vi "Get 2614B value.vi"(11 "输出簇输入":T1 {"Instrument"."Input (0:A)" items=["A", "B"]; "Instrument"."Heater Output (1:1)" items=["1"=1, "2"=2]; "SR830+6221"."Reserve 4" items=["Auto Reserve"=-1, "High Reserve"=0, "Normal"=1, "Low Noise"=2]; "SR830+6221"."Reserve 3" items=["Auto Reserve"=-1, "High Reserve"=0, "Normal"=1, "Low Noise"=2]; "SR830+6221"."Reserve 2" items=["Auto Reserve"=-1, "High Reserve"=0, "Normal"=1, "Low Noise"=2]; "SR830+6221"."Reserve 1" items=["Auto Reserve"=-1, "High Reserve"=0, "Normal"=1, "Low Noise"=2]; "SR830+6221"."source" items=["SR830 1", "SR830 2", "SR830 3", "SR830 4"]}) -> (3 "数组":string[](array[string]))   [LabVIEW 2019, in "Get value.lvlib"]
uses:
  config.ctl
  <vilib>/NI/Modbus Library/API/Master/Modbus Master.lvclass
  initialize.ctl
  Instrument.ctl
  Instrument Type.ctl
  lib/QDInstrument.dll
  335 state.ctl
  SubVI/limit.ctl
  9T mag field stauts.ctl
  warning.ctl
  lib/Keithley 2600 Series/Public/Data/Read Measurement (Current and Voltage).vi
  SubVI/Get value.lvlib
  lib/Keithley 2600 Series/Keithley 2600 Series.lvlib
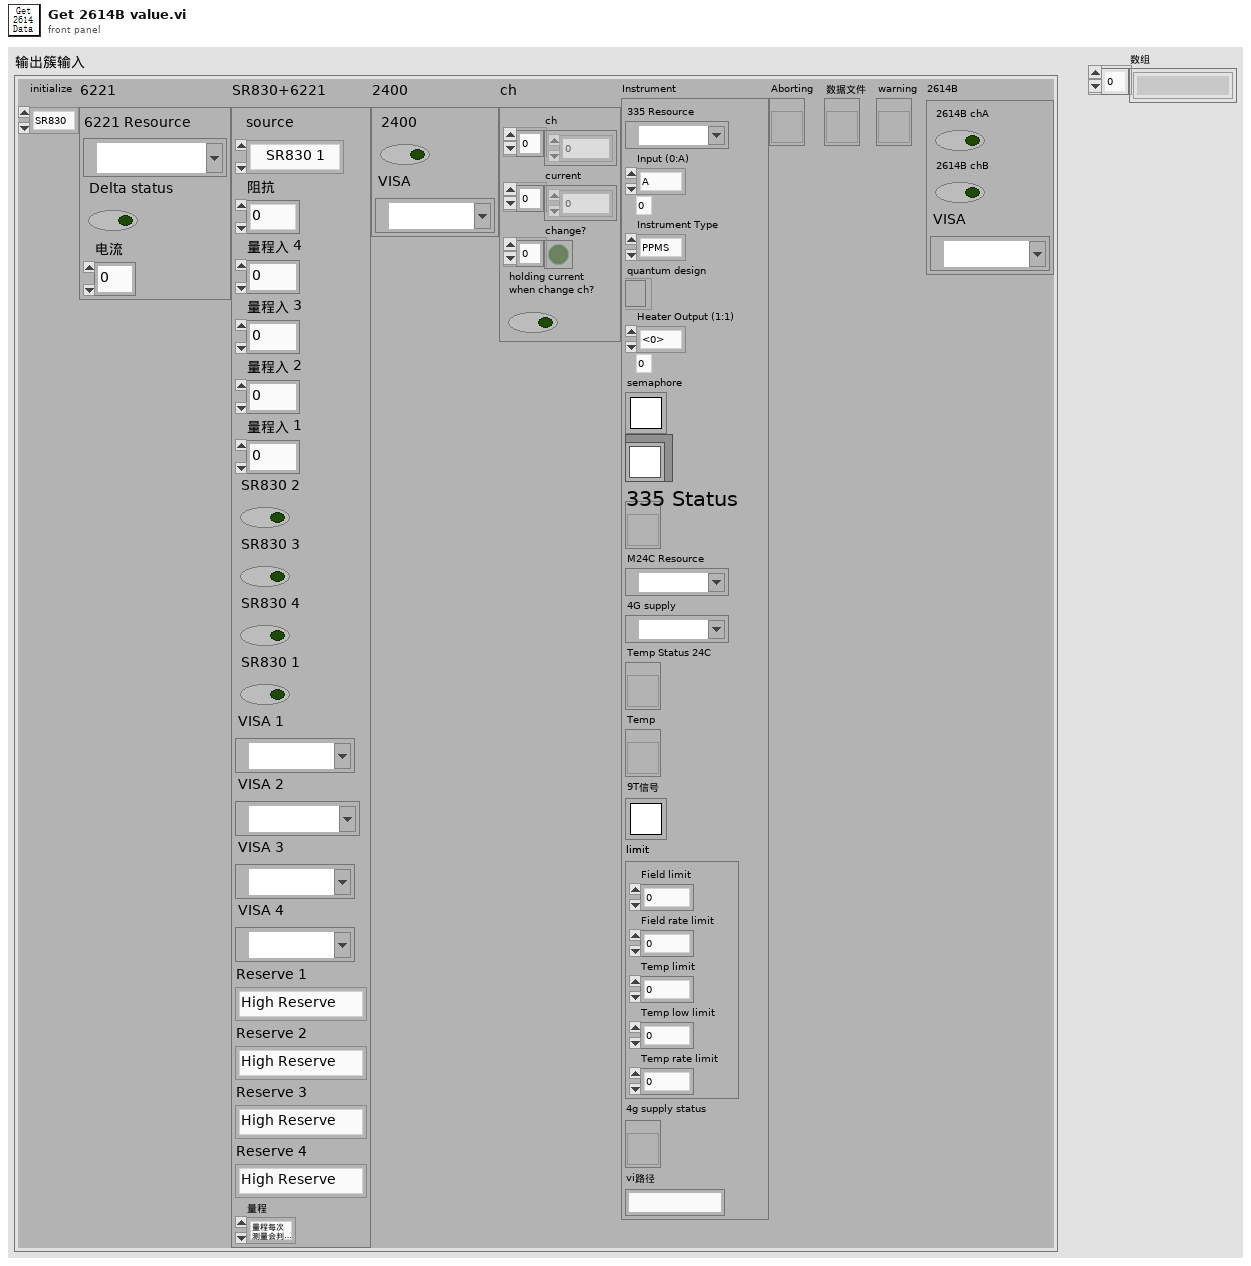
[diagram p1: front panel]
types:
  T1 = typedef "config.ctl" = cluster{"initialize":T2, "6221":cluster{"6221 Resource":refnum<visa-resource-name>, "Delta status":bool, "电流":dbl}, "SR830+6221":cluster{"source":u16, "阻抗":dbl, "量程入 4":i32, "量程入 3":i32, "量程入 2":i32, "量程入 1":i32, "SR830 2":bool, "SR830 3":bool, "SR830 4":bool, "SR830 1":bool, "VISA 1":refnum<visa-resource-name>, "VISA 2":refnum<visa-resource-name>, "VISA 3":refnum<visa-resource-name>, "VISA 4":refnum<visa-resource-name>, "Reserve 1":i16, "Reserve 2":i16, "Reserve 3":i16, "Reserve 4":i16, "量程":enum16{"量程每次测量会判定", "量程不变为设定值"}}, "2400":cluster{"2400":bool, "VISA":refnum<visa-resource-name>}, "ch":cluster{"ch":i32[], "current":dbl[], "change?":bool[], "holding current\nwhen change ch?":bool}, "Instrument":T3, "Aborting":refnum<vi>, "数据文件":refnum<vi>, "warning":refnum<vi>, "2614B":cluster{"2614B chA":bool, "2614B chB":bool, "VISA":refnum<visa-resource-name>}}
  T2 = typedef "initialize.ctl" = enum16{"SR830", "keithley6221-SR830", "Delta", "Delta-tunnelling", "keithley6221-2182-DC"}
  T3 = typedef "Instrument.ctl" = cluster{"335 Resource":refnum<visa-resource-name>, "Input (0:A)":u16, "Instrument Type":T4, "quantum design":refnum<k24>, "Heater Output (1:1)":u16, "semaphore":T5, "TCP master instance":refnum<class "Modbus Master.lvclass">, "335 Status":refnum<vi>, "M24C Resource":refnum<visa-resource-name>, "4G supply":refnum<visa-resource-name>, "Temp Status 24C":refnum<vi>, "Temp":refnum<vi>, "9T信号":T5, "limit":T6, "4g supply status":refnum<vi>, "vi路径":string}
  T4 = typedef "Instrument Type.ctl" = enum16{"PPMS", "VersaLab", "DynaCool", "SVSM", "PPMS-Rotate", "Lakeshore335", "9T mag"}
  T5 = typedef "Semaphore RefNum" = refnum<k1>
  T6 = typedef "limit.ctl" = cluster{"Field limit":dbl, "Field rate limit":dbl, "Temp limit":dbl, "Temp low limit":dbl, "Temp rate limit ":dbl}
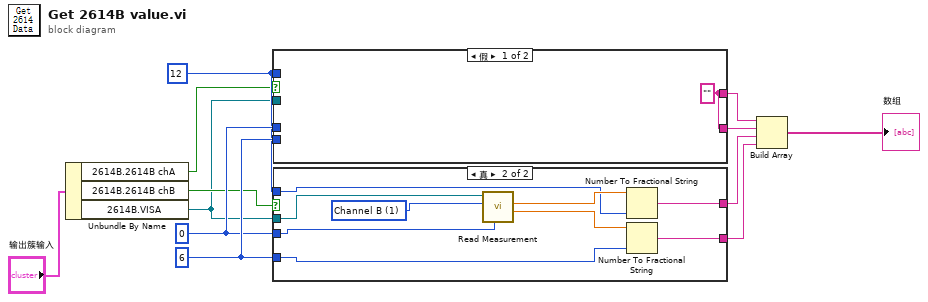
[diagram p0: block diagram]
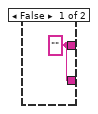
[diagram p2: hidden frame]
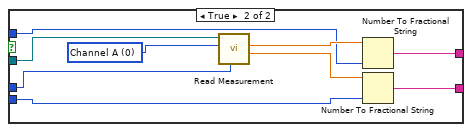
[diagram p3: hidden frame]
diagram:
  w6 = 0 ("Wait Time (10 S)")
  w5 = i16 12 ("精度(6)")
  w7 = i16 6 ("精度(6)")
  n1 = Unbundle By Name("输出簇输入") -> ("2614B.2614B chA"=w2:bool, "2614B.2614B chB"=w4:bool, "2614B.VISA"=w3:refnum<visa-resource-name>)
  n2 = case shown="假" w2 {
    tunnel: w3 -> [_ w22]
    tunnel: w5 -> [_ w19]
    tunnel: w6 -> [_ w18]
    tunnel: w7 -> [_ w16]
    tunnel: [w13 w15] -> w8
    tunnel: [w13 w14] -> w9
    frame False {
      w13 = ""
    }
    frame True {
      w21 = 0 items=["Channel A", "Channel B"] ("Source Measure Unit Channel (0: Channel A)")
      n3 = call-poly "Read Measurement.vi"("Wait Time (10 S)"=w18, "Source Measure Unit Channel (0: Channel A)"=w21, "VISA resource name"=w22) -> ("Last Voltage (V)"=w17:dbl, "Last Current (A)"=w20:dbl)  [unwired: 3 in, 4 out]
      n4 = Number To Fractional String(number=w20, precision (6)=w19) -> (F-format string=w15:string)  [unwired: 2 in]
      n5 = Number To Fractional String(number=w17, precision (6)=w16) -> (F-format string=w14:string)  [unwired: 2 in]
    }
  }
  n6 = case shown="真" w4 {
    tunnel: w3 -> [_ w32]
    tunnel: w7 -> [_ w28]
    tunnel: w5 -> [_ w27]
    tunnel: w6 -> [_ w26]
    tunnel: [w23 w25] -> w10
    tunnel: [w23 w24] -> w11
    frame False {
      w23 = ""
    }
    frame True {
      w31 = 1 items=["Channel A", "Channel B"] ("Source Measure Unit Channel (0: Channel A)")
      n7 = call-poly "Read Measurement.vi"("Wait Time (10 S)"=w26, "Source Measure Unit Channel (0: Channel A)"=w31, "VISA resource name"=w32) -> ("Last Voltage (V)"=w29:dbl, "Last Current (A)"=w30:dbl)  [unwired: 3 in, 4 out]
      n8 = Number To Fractional String(number=w30, precision (6)=w27) -> (F-format string=w25:string)  [unwired: 2 in]
      n9 = Number To Fractional String(number=w29, precision (6)=w28) -> (F-format string=w24:string)  [unwired: 2 in]
    }
  }
  n10 = Build Array(w8, w9, w10, w11) -> (→"数组":string[])
